vi "保存 ini.vi"() -> ()   [LabVIEW 2016]
uses:
  <vilib>/Utility/config.llb/Write Key (Double).vi
  <vilib>/Utility/config.llb/Read Key (Double).vi
  <vilib>/Utility/config.llb/NI_LVConfig.lvlib
panel:
  in  "打开位置":path
  in  "读取":bool
  in  "保存":bool
  in  "保存位置":path
  in  "电压 下限":dbl
  in  "电流 下限":dbl
  in  "电压 上限":dbl
  in  "电流 上限":dbl
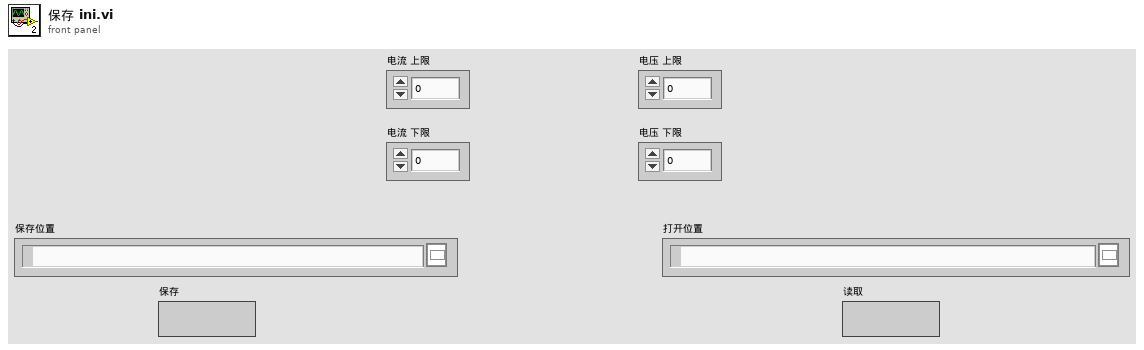
[diagram p1: front panel]
types:
  T1 = typedef "NI_LVConfig.lvlib/Config Data RefNum.ctl" = refnum<k1>
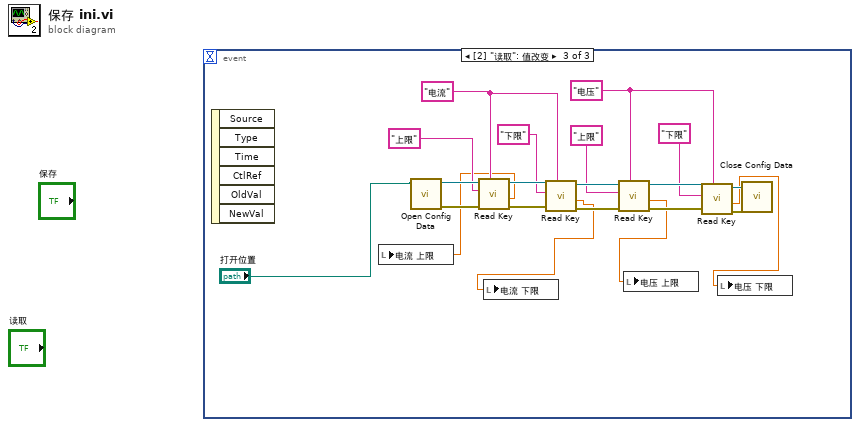
[diagram p0: block diagram]
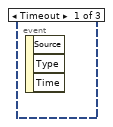
[diagram p2: hidden frame]
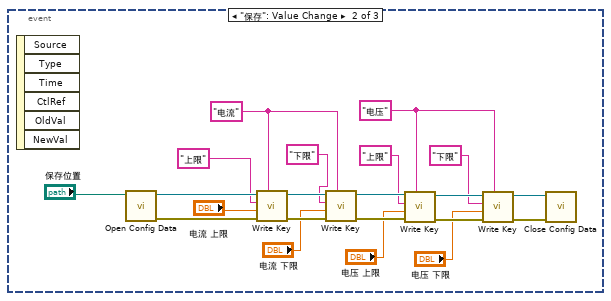
[diagram p3: hidden frame]
diagram:
  n1 = event shown="[2] \"读取\": 值改变" {
    selector: _ -> [_ _ _]
    dyn-events: _ -> [_ _ _]
    timeout: _ -> [_ _ _]
    event Timeout {
      n2 = event-data() -> ()  [unwired: 1 in, 3 out]
    }
    event "保存": Value Change {
      w5 = "电压"
      w9 = "电流"
      n3 = event-data() -> ()  [unwired: 1 in, 6 out]
      n4 = call <vilib>:"Open Config Data.vi"("configuration file path"="保存位置") -> ("error out"=w18:errorcluster, "refnum"=w20:T1)  [unwired: 8 in, 1 out]
      n5 = call-poly <vilib>:"Write Key.vi"("section"=w9, "error in (no error)"=w18, "value"="电流 上限", "key"="上限", "refnum"=w20) -> ("error out"=w17:errorcluster, "refnum out"=w16:T1)  [unwired: 4 in, 1 out]
      n6 = call-poly <vilib>:"Write Key.vi"("section"=w9, "error in (no error)"=w17, "value"="电流 下限", "key"="下限", "refnum"=w16) -> ("error out"=w15:errorcluster, "refnum out"=w14:T1)  [unwired: 4 in, 1 out]
      n7 = call-poly <vilib>:"Write Key.vi"("section"=w5, "error in (no error)"=w15, "value"="电压 上限", "key"="上限", "refnum"=w14) -> ("error out"=w13:errorcluster, "refnum out"=w12:T1)  [unwired: 4 in, 1 out]
      n8 = call-poly <vilib>:"Write Key.vi"("section"=w5, "error in (no error)"=w13, "value"="电压 下限", "key"="下限", "refnum"=w12) -> ("error out"=w10:errorcluster, "refnum out"=w11:T1)  [unwired: 4 in, 1 out]
      n9 = call <vilib>:"Close Config Data.vi"("error in (no error)"=w10, "refnum"=w11) -> ()  [unwired: 8 in, 2 out]
    }
    event "读取": Value Change {
      w29 = "电压"
      w30 = "电流"
      n10 = event-data() -> ()  [unwired: 1 in, 6 out]
      n11 = call <vilib>:"Open Config Data.vi"("configuration file path"="打开位置") -> ("error out"=w42:errorcluster, "refnum"=w41:T1)  [unwired: 8 in, 1 out]
      n12 = call-poly <vilib>:"Read Key.vi"("section"=w30, "error in (no error)"=w42, "key"="上限", "refnum"=w41) -> ("error out"=w40:errorcluster, "value"=w25:dbl, "refnum out"=w39:T1)  [unwired: 4 in, 1 out]
      n13 = local write "电流 上限"(w25) -> ()
      n14 = call-poly <vilib>:"Read Key.vi"("section"=w30, "error in (no error)"=w40, "key"="下限", "refnum"=w39) -> ("error out"=w38:errorcluster, "value"=w24:dbl, "refnum out"=w37:T1)  [unwired: 4 in, 1 out]
      n15 = local write "电流 下限"(w24) -> ()
      n16 = call-poly <vilib>:"Read Key.vi"("section"=w29, "error in (no error)"=w38, "key"="上限", "refnum"=w37) -> ("error out"=w36:errorcluster, "value"=w22:dbl, "refnum out"=w35:T1)  [unwired: 4 in, 1 out]
      n17 = local write "电压 上限"(w22) -> ()
      n18 = call-poly <vilib>:"Read Key.vi"("section"=w29, "error in (no error)"=w36, "key"="下限", "refnum"=w35) -> ("error out"=w34:errorcluster, "value"=w23:dbl, "refnum out"=w33:T1)  [unwired: 4 in, 1 out]
      n19 = local write "电压 下限"(w23) -> ()
      n20 = call <vilib>:"Close Config Data.vi"("error in (no error)"=w34, "refnum"=w33) -> ()  [unwired: 8 in, 2 out]
    }
  }
